vi "OnDataChange.vi"(0 "GRMActor in":refnum<class "QPDController.lvclass">, 1 "DataExchange":T1, 3 "error in (no error)":errorcluster) -> (7 "GRMActor out":refnum<class "QPDController.lvclass">, 10 "error out":errorcluster)   [LabVIEW 2020, in "QPDController.lvlib" / "QPDController.lvclass"]
uses:
  QPDController.lvclass
  C:/Program Files/National Instruments/LabVIEW 2020/vi.lib/ActorFramework/Actor/Actor.lvclass
  Model/Hardware Abstraction Layer/Component/Device/Device/DataExchange.ctl
  <vilib>/ActorFramework/Actor/Actor.lvclass/Actor.ctl
  Interface/DataListener Messages/OnDataChange Msg/OnDataChange Msg.lvclass/OnDataChange Msg.ctl
  <vilib>/ActorFramework/Message Enqueuer/Message Enqueuer.lvclass/Message Enqueuer.ctl
  QPDExchangeData.ctl
  QPDController.lvclass/QPDController.ctl
  <vilib>/ActorFramework/Message Enqueuer/Enqueue.vi
  Interface/DataListener Messages/OnDataChange Msg/OnDataChange Msg.lvclass
  C:/Program Files/National Instruments/LabVIEW 2020/vi.lib/ActorFramework/Message/Message.lvclass
  <vilib>/ActorFramework/Message Priority Queue/Priority Enqueue.vi
  Model/Hardware Abstraction Layer/Component/GenericActor/GenericActor/GenericController.lvclass
  <vilib>/ActorFramework/Actor/Actor.lvclass
  QPDController.lvlib
  Interface/DataListener/DataListener.lvclass
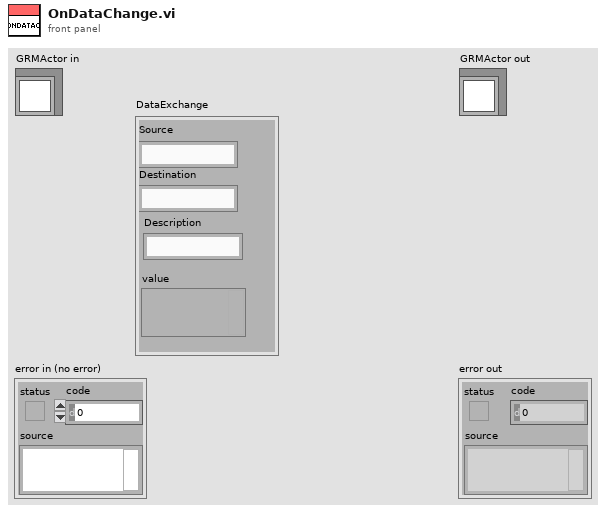
[diagram p1: front panel]
types:
  T1 = typedef "DataListener.lvclass/DataExchange.ctl" = cluster{"Source":string, "Destination":string, "Description":string, "value":variant}
  T2 = typedef "QPDController.lvlib/QPDExchangeData.ctl" = cluster{"Kd":dbl, "Sampling Rate":dbl, "Ki":dbl, "Kp":dbl}
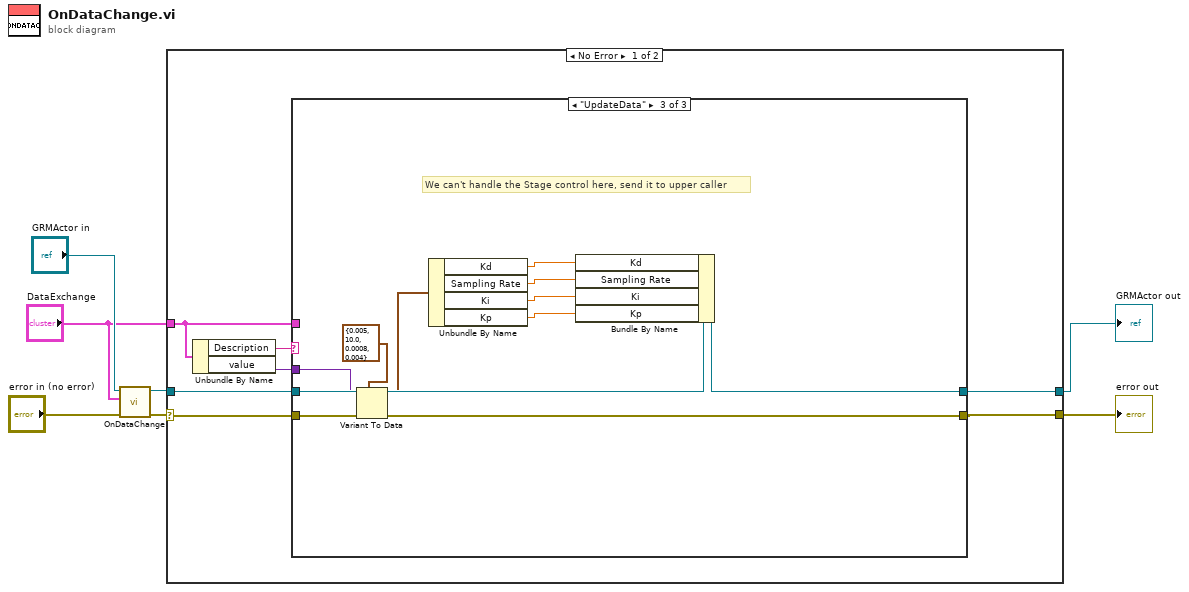
[diagram p0: block diagram]
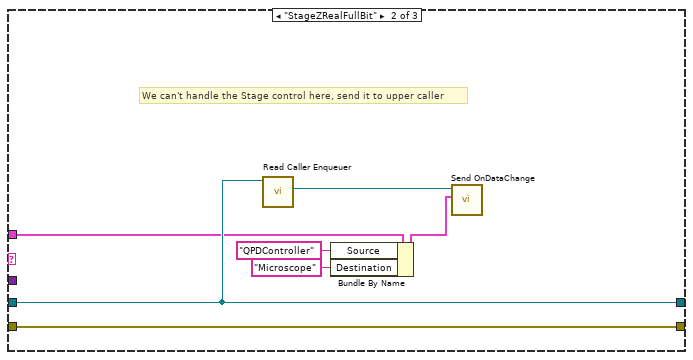
[diagram p3: hidden frame]
diagram:
  n1 = call-parent "OnDataChange.vi"("GRMActor in"="GRMActor in", "DataExchange"="DataExchange", "error in (no error)"="error in (no error)") -> ("GRMActor out"=w4:refnum<class "QPDController.lvclass">, "error out"=w5:errorcluster)  [unwired: 6 in]
  n2 = case shown="No Error" w5 {
    selector: w5 -> [w11 w35]
    tunnel: [w10 w35] -> w1
    tunnel: [w9 w36] -> w2
    tunnel: w4 -> [w12 w36]
    tunnel: "DataExchange" -> [w8 _]
    frame No Error {
      n3 = Unbundle By Name(w8) -> ("Description"=w14:string, "value"=w13:variant)
      n4 = case shown="\"UpdateData\"" w14 {
        tunnel: w13 -> [_ _ w31]
        tunnel: [w16 w22 w29] -> w9
        tunnel: w12 -> [w16 w22 w33]
        tunnel: [w15 w23 w32] -> w10
        tunnel: w11 -> [w15 w23 w34]
        tunnel: w8 -> [_ w20 _]
        frame Default {
        }
        frame "StageZRealFullBit" {
          # "We can't handle the Stage control here, send it to upper caller"
          n5 = call <vilib>:"Read Caller Enqueuer.vi"("Actor"=w22) -> ("Caller Enqueuer"=w21:refnum<class "Message Enqueuer.lvclass">)  [unwired: 10 in]
          n6 = Bundle By Name(cluster=w20, "Source"="QPDController", "Destination"="Microscope") -> (w19:T1)
          n7 = call "Send OnDataChange.vi"("DataExchange"=w19, "Message Enqueuer"=w21) -> ()  [unwired: 8 in, 2 out]
        }
        frame "UpdateData" {
          # "We can't handle the Stage control here, send it to upper caller"
          n8 = Variant To Data(error in=w34, type=T2 {"Kd"=0.005, "Sampling Rate"=10.0, "Ki"=0.0008, "Kp"=0.004} ("Cluster"), Variant=w31) -> (data=w28:T2, error out=w32:errorcluster)
          n9 = Unbundle By Name(w28) -> ("Kd"=w27:dbl, "Sampling Rate"=w26:dbl, "Ki"=w25:dbl, "Kp"=w24:dbl)
          n10 = Bundle By Name(cluster=w33, "Kd"=w27, "Sampling Rate"=w26, "Ki"=w25, "Kp"=w24) -> (w29:refnum<class "QPDController.lvclass">)
        }
      }
    }
    frame Error {
    }
  }
  "error out" <- w1
  "GRMActor out" <- w2
